vi "UTILITY Find Configuration File.vi"(7 "Read Default Path":bool, 8 "Error In":errorcluster, 11 "File Locations In":T1) -> (0 "Error Out":errorcluster, 2 "Full System Path (String)":string, 3 "File Locations Out":T1)   [LabVIEW 2016]
uses:
  Save File/File Setup (Public)/Type Definition/Save File DOE File Path Control.ctl
  Save File/File Setup (Public)/Type Definition/Save File DOE Data Save Filepaths.ctl
  <vilib>/Utility/file.llb/Read Delimited Spreadsheet (string).vi
  Save File/File Setup.lvlib
panel:
  out "all rows":string[][](array[string])
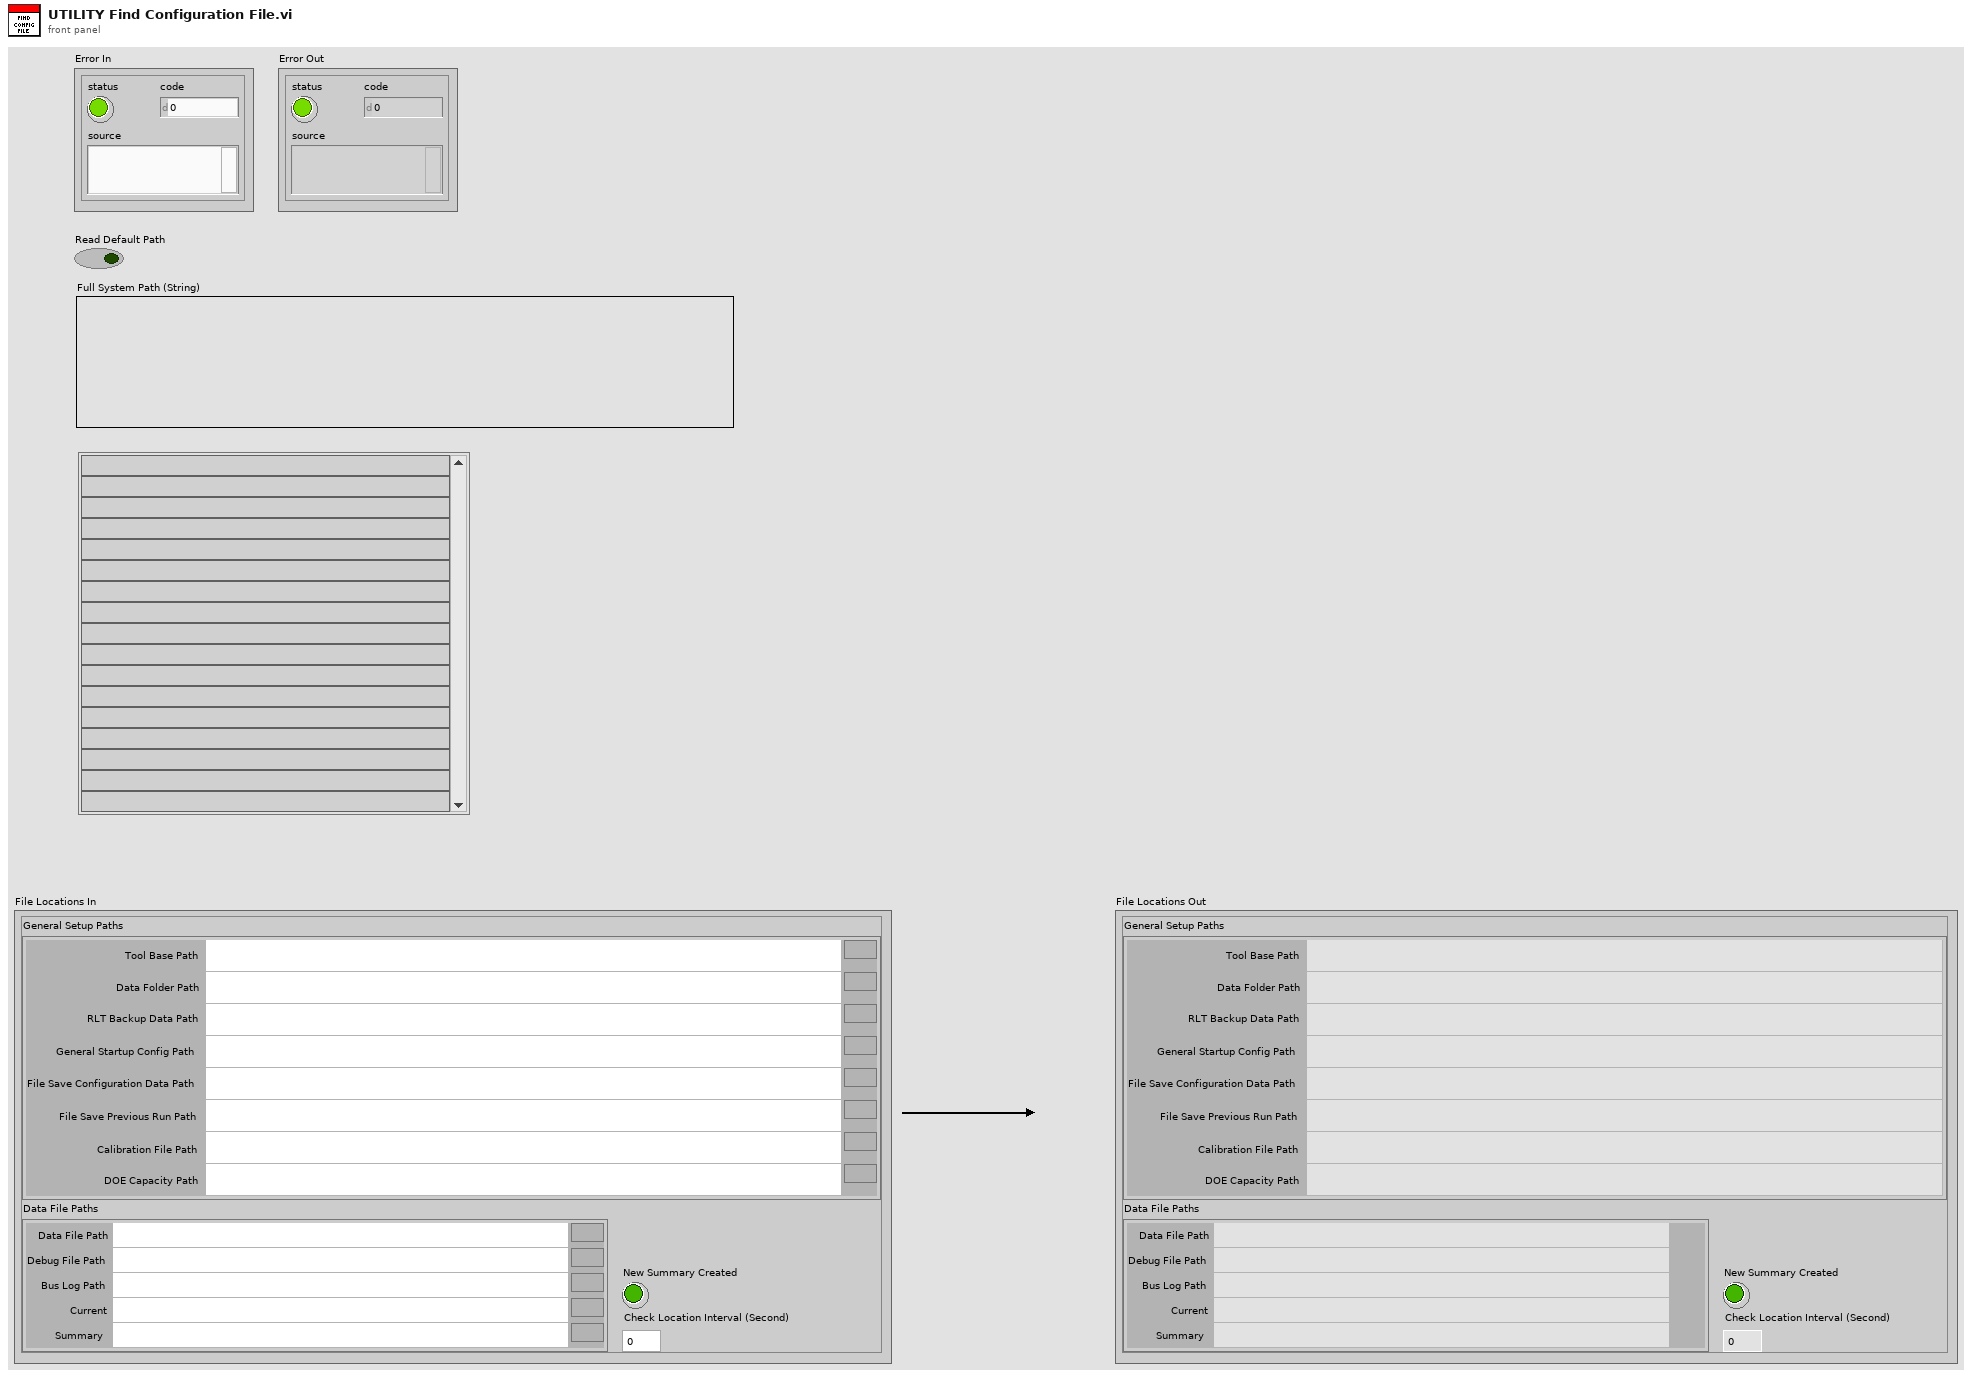
[diagram p1: front panel]
types:
  T1 = typedef "File Setup.lvlib/Save File DOE File Path Control.ctl" = cluster{"General Setup Paths":cluster{"Calibration File Path":path, "DOE Capacity Path":path, "Data Folder Path":path, "RLT Backup Data Path":path, "Tool Base Path":path, "General Startup Config Path":path, "File Save Previous Run Path":path, "File Save Configuration Data Path":path}, "Data File Paths":T2, "New Summary Created":bool, "Check Location Interval (Second)":i32}
  T2 = typedef "File Setup.lvlib/Save File DOE Data Save Filepaths.ctl" = cluster{"Data File Path":path, "Debug File Path":path, "Bus Log Path":path, "Current":path, "Summary":path}
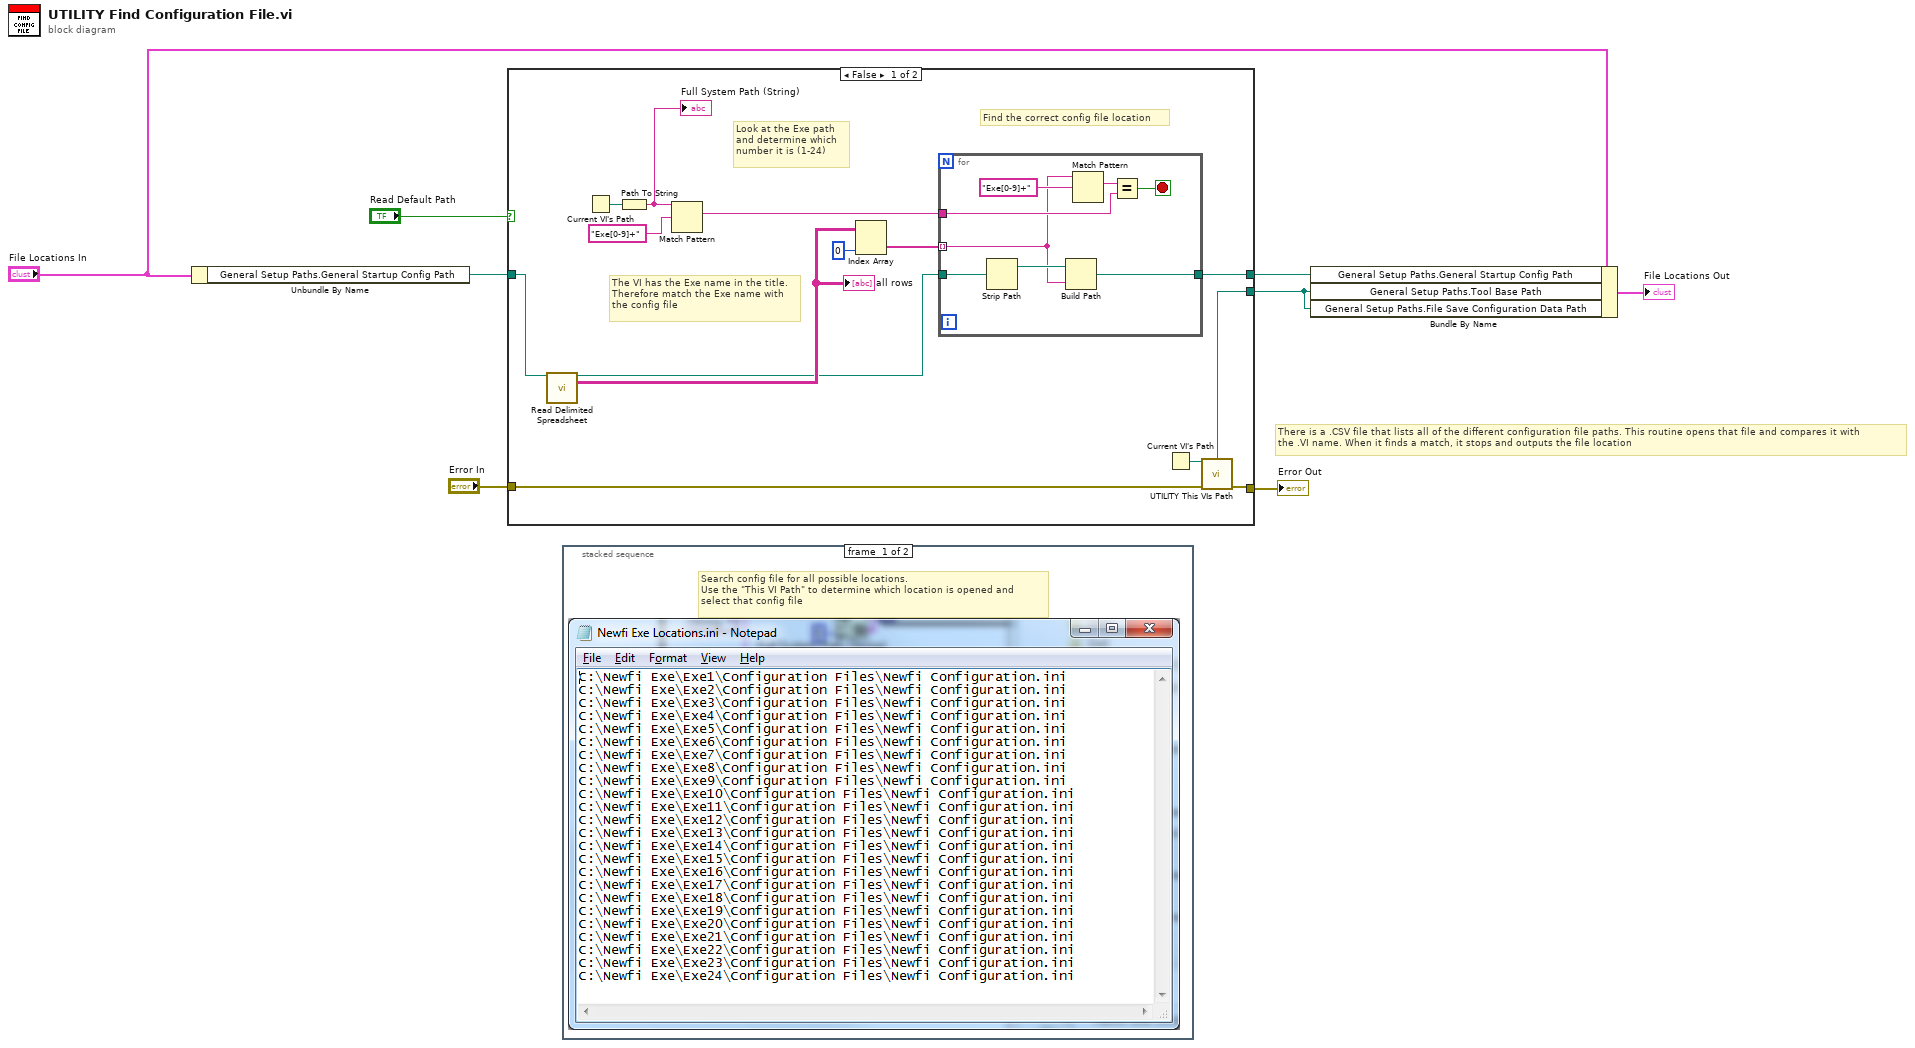
[diagram p0: block diagram]
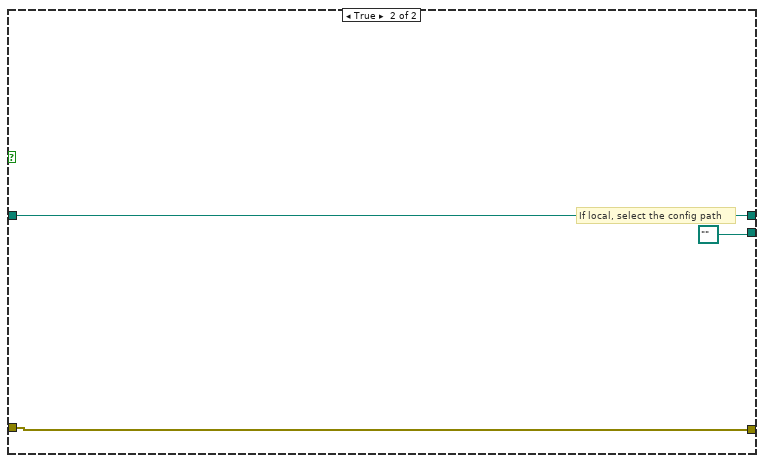
[diagram p3: hidden frame]
diagram:
  # "There is a .CSV file that lists all of the different configuration file paths. This routine opens that file and compares it with\nthe .VI name. When it finds a match, it stops and outputs the file location"
  n1 = Unbundle By Name("File Locations In") -> ("General Setup Paths.General Startup Config Path"=w6:path)
  n2 = case shown="False" "Read Default Path" {
    tunnel: [w15 w32] -> w4
    tunnel: w6 -> [w20 w32]
    tunnel: "Error In" -> [w13 w33]
    tunnel: [w12 w33] -> w7
    tunnel: [w11 path "" ("Folder Path")] -> w1
    frame False {
      # "The VI has the Exe name in the title.\nTherefore match the Exe name with\nthe config file"
      # "Find the correct config file location"
      # "Look at the Exe path\nand determine which\nnumber it is (1-24)"
      n3 = call-poly <vilib>:"Read Delimited Spreadsheet.vi"("file path (dialog if empty)"=w20) -> ("new file path (Not A Path if cancelled)"=w9:path, "all rows"=w10:string[][])  [unwired: 9 in, 4 out]
      "all rows" <- w10
      n4 = Current VI's Path() -> (path=w17:path)
      n5 = Path To String(path=w17) -> (string=w19:string)
      "Full System Path (String)" <- w19
      n6 = Match Pattern(string=w19, regular expression="Exe[0-9]+") -> (match substring=w16:string)  [unwired: 1 in, 3 out]
      n7 = Index Array(array=w10, index (col)=0 ("disabled index (col)")) -> (element=w22:string[])  [unwired: 1 in]
      n8 = for {
        tunnel: w22 -> [w24] mode=indexing
        tunnel: [w23] -> w15
        tunnel: w16 -> [w28]
        tunnel: w9 -> [w26]
        stop <- w27 stop-if-true
        n9 = Strip Path(path=w26) -> (stripped path=w25:path)  [unwired: 1 out]
        n10 = Build Path(base path=w25, name or relative path=w24) -> (appended path=w23:path)
        n11 = Match Pattern(string=w24, regular expression="Exe[0-9]+") -> (match substring=w29:string)  [unwired: 1 in, 3 out]
        n12 = Equal?(x=w29, y=w28) -> (x = y?=w27:bool)
      }
      n13 = Current VI's Path() -> (path=w14:path)
      n14 = call "UTILITY This VIs Path.vi"("path"=w14, "error in (no error)"=w13) -> ("Folder Path"=w11:path, "error out"=w12:errorcluster)  [unwired: 7 in, 5 out]
    }
    frame True {
      # "If local, select the config path"
    }
  }
  "Error Out" <- w7
  n15 = stacked-sequence {
    frame #0 {
      # "Search config file for all possible locations.\nUse the \"This VI Path\" to determine which location is opened and \nselect that config file"
    }
    frame #1 {
    }
  }
  n16 = Bundle By Name(cluster="File Locations In", "General Setup Paths.General Startup Config Path"=w4, "General Setup Paths.Tool Base Path"=w1, "General Setup Paths.File Save Configuration Data Path"=w1) -> (→"File Locations Out":T1)
